vi "Generate Sequence (RNN).vi"(0 "sample length":u64, 5 "dimension":u64, 7 "index seed":u64, 9 "hidden state (in)":T1 format="%_8f", 11 "params":T2) -> (6 "sequence out":u64[](array[numeric]), 10 "hidden state (out)":T1 format="%_8f")   [LabVIEW 2014]
uses:
  <vilib>/Analysis/Matrix/Datatypes/RealMatrix.ctl
  <vilib>/Analysis/Matrix/NI_Matrix.lvlib
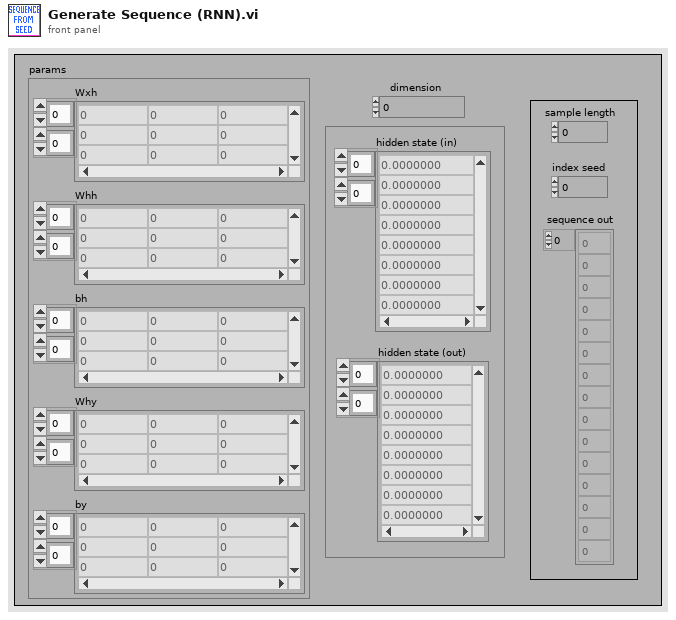
[diagram p1: front panel]
types:
  T1 = typedef "NI_Matrix.lvlib/RealMatrix.ctl" = dbl[][]
  T2 = cluster{"Wxh":T1, "Whh":T1, "bh":T1, "Why":T1, "by":T1}
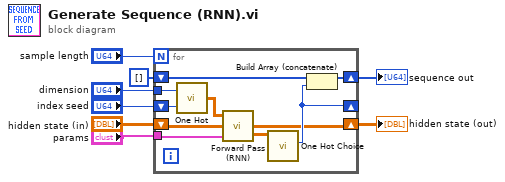
[diagram p0: block diagram]
diagram:
  n1 = for {
    N: "sample length" -> [_]
    shift-right: [w17] -> w7
    shift-left: u64[] [] -> [w16]
    shift-right: [w15] -> _
    shift-left: "index seed" -> [w11]
    shift-right: [w13] -> w8
    shift-left: "hidden state (in)" -> [w12]
    tunnel: "params" -> [w14]
    tunnel: "dimension" -> [w10]
    n2 = call "One Hot.vi"("hot index"=w11, "length"=w10) -> ("One hot vector"=w9:T1)
    n3 = call "Forward Pass (RNN).vi"("params"=w14, "h[t-1]"=w12, "x[t]"=w9) -> ("p[t]"=w18:T1, "h[t]"=w13:T1)
    n4 = call "One Hot Choice.vi"("Probabilities"=w18) -> ("hot index"=w15:u64)  [unwired: 8 in, 2 out]
    n5 = Build Array (concatenate)(w16, w15) -> (w17:u64[])
  }
  "hidden state (out)" <- w8
  "sequence out" <- w7
